vi "FGEN_CLOSED.vi"(8 "error in":errorcluster caption="error in (no error)", 11 "instrument handle":refnum<k15>="PXI1Slot2") -> (0 "error out":errorcluster)   [LabVIEW 2013]
doc: "Configures and runs National Instruments signal generators using NI-FGEN in Standard Function output mode.\n\nYou must place at least two NI-FGEN Express (Standard Functions) VIs on the block diagram for successful function generation. Select <B>Start generation</B> for the Generation Mode in the first Express VI to start the continuous function generation. Select <B>Stop generation</B> for the Generation Mode in the final Express VI to abort function generation and close the NI-FGEN device handle.\n--------------------\n\nThis Express VI is configured as follows:\n\nDevice: PXI1Slot2 (PXI-5402)\nChannel 0\n - Disable output on close: False"
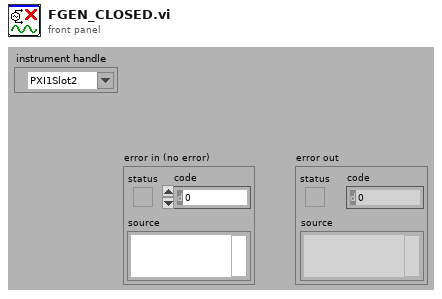
[diagram p1: front panel]
types:
  T1 = cluster{"channel name":string, "output enable":bool}[]
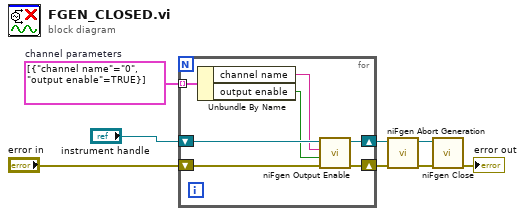
[diagram p0: block diagram]
diagram:
  w1 = T1 [{"channel name"="0", "output enable"=TRUE}]  # channel parameters
  n1 = for {
    shift-right: [w14] -> w6
    shift-left: "error in" -> [w15]
    shift-right: [w12] -> w3
    shift-left: "instrument handle" -> [w13]
    tunnel: w1 -> [w11] mode=indexing
    n2 = Unbundle By Name(w11) -> ("channel name"=w10:string, "output enable"=w9:bool)
    n3 = call <instrlib>:"niFgen Output Enable.vi"("error in (no error)"=w15, "Output Enable (default: True)"=w9, "Channel Name"=w10, "Instrument Handle"=w13) -> ("error out"=w14:errorcluster, "Instrument Handle Out"=w12:refnum<k15>)  [unwired: 6 in]
  }
  n4 = call <instrlib>:"niFgen Abort Generation.vi"("error in (no error)"=w6, "Instrument Handle"=w3) -> ("error out"=w5:errorcluster, "Instrument Handle Out"=w2:refnum<k15>)  [unwired: 8 in]
  n5 = call <instrlib>:"niFgen Close.vi"("error in (no error)"=w5, "Instrument Handle"=w2) -> ("error out"=→"error out":errorcluster)  [unwired: 9 in]
